vi "JSON Reponse.vi"() -> ()   [LabVIEW 2020, in "obs-scratch.lvlib"]
uses:
  obs-scratch.lvlib
  obs-websocket/GetSceneItemTransform/GetSceneItemTransform.lvclass
  C:/dev/lv20CE/relink/lv-obs-websocket/obs-websocket/Client Message/Client Message.lvclass
  obs-websocket/OBS/OBS.lvclass
  <vilib>/JDP Science/JSONtext/JSONtext.lvlib
  C:/dev/lv20CE/relink/lv-obs-websocket/obs-websocket/Request/Request.lvclass
  C:/dev/lv20CE/relink/lv-obs-websocket/obs-websocket/Message/Message.lvclass
  C:/dev/lv20CE/relink/lv-obs-websocket/obs-websocket/GetSceneItemTransform/GetSceneItemTransform.lvclass
panel:
  in  "Scale":dbl(slide) scale=0.1..5.0
  in  "Rotation":dbl min=-180.0 max=180.0 format="%0.2f"
  in  "stop":bool
  out "JSON Response":string
  out "error out":errorcluster
  in  "Password":string="44S4aN6PpCHpVM4Y"
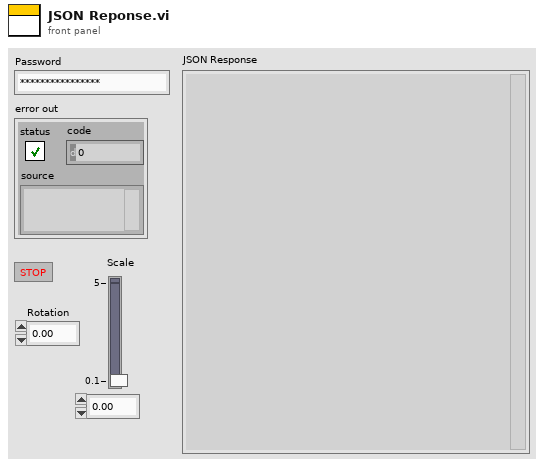
[diagram p1: front panel]
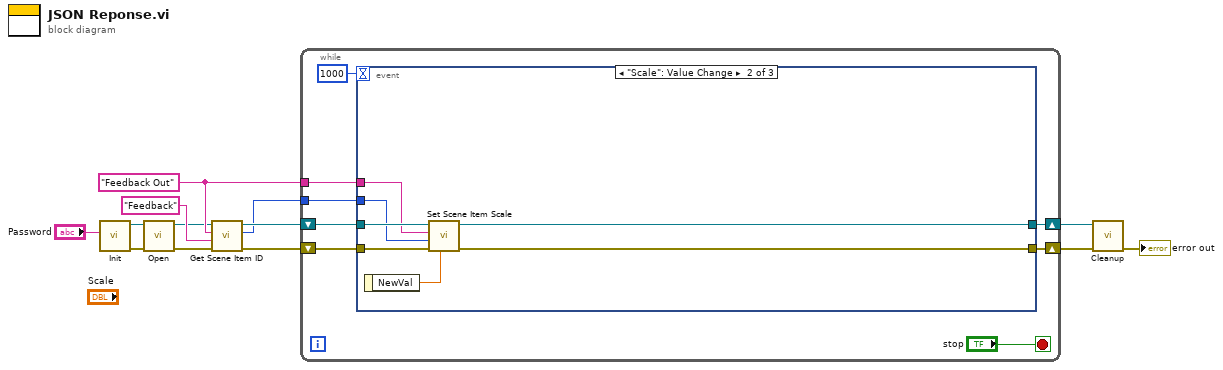
[diagram p0: block diagram]
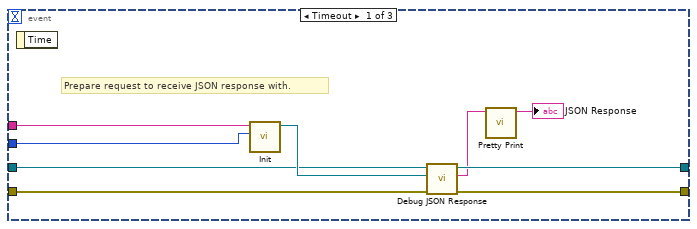
[diagram p2: hidden frame]
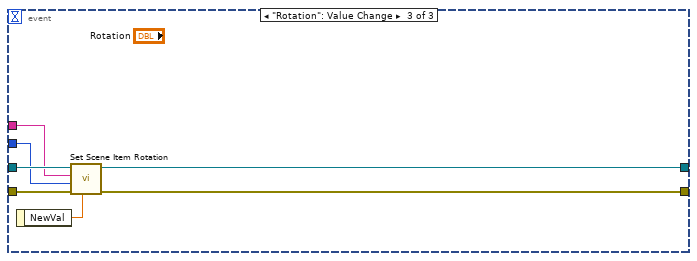
[diagram p3: hidden frame]
diagram:
  w6 = "Feedback Out" ("Scene Name")
  n1 = call "Init.vi"("Password (None)"="Password") -> ("error out"=w12:errorcluster, "OBS out"=w13:refnum<class "OBS.lvclass">)  [unwired: 9 in]
  n2 = call "Open.vi"("error in (no error)"=w12, "OBS in"=w13) -> ("error out"=w4:errorcluster, "OBS out"=w5:refnum<class "OBS.lvclass">)  [unwired: 8 in]
  n3 = call "Get Scene Item ID.vi"("error in (no error)"=w4, "Source Name"="Feedback" ("Scene Name"), "Scene Name"=w6, "OBS in"=w5) -> ("error out"=w3:errorcluster, "Scene Item ID"=w1:i32, "OBS out"=w2:refnum<class "OBS.lvclass">)  [unwired: 5 in]
  n4 = while {
    shift-right: [w18] -> w9
    shift-left: w2 -> [w21]
    shift-right: [w19] -> w10
    shift-left: w3 -> [w20]
    tunnel: w6 -> [w15]
    tunnel: w1 -> [w14]
    stop <- "stop" stop-if-true
    n5 = event shown="[1] \"Scale\": Value Change" {
      selector: _ -> [_ _ _]
      dyn-events: _ -> [_ _ _]
      timeout: 1000 -> [_ _ _]
      tunnel: w21 -> [w23 w37 w44]
      tunnel: w20 -> [w22 w36 w43]
      tunnel: [w29 w31 w38] -> w19
      tunnel: [w28 w32 w39] -> w18
      tunnel: w15 -> [w25 w33 w41]
      tunnel: w14 -> [w24 w34 w40]
      event Timeout {
        # "Prepare request to receive JSON response with."
        n6 = event-data() -> ()  [unwired: 1 in, 1 out]
        n7 = call "Init.vi"("Scene Item ID"=w24, "Scene Name"=w25) -> ("GetSceneItemTransform out"=w30:refnum<class "GetSceneItemTransform.lvclass">)  [unwired: 8 in, 1 out]
        n8 = call "Debug JSON Response.vi"("error in (no error)"=w22, "Client Message"=w30, "OBS in"=w23) -> ("error out"=w29:errorcluster, "JSON Response"=w27:string, "OBS out"=w28:refnum<class "OBS.lvclass">)  [unwired: 5 in, 1 out]
        n9 = call <vilib>:"Pretty Print.vi"("JSON"=w27) -> ("<JSON>"=→"JSON Response":string)  [unwired: 8 in, 2 out]
      }
      event "Scale": Value Change {
        n10 = event-data() -> ("NewVal"=w35:dbl)  [unwired: 1 in]
        n11 = call "Set Scene Item Scale.vi"("Scale"=w35, "error in (no error)"=w36, "Scene Item ID"=w34, "Scene Name"=w33, "OBS in"=w37) -> ("error out"=w31:errorcluster, "OBS out"=w32:refnum<class "OBS.lvclass">)  [unwired: 5 in]
      }
      event "Rotation": Value Change {
        n12 = event-data() -> ("NewVal"=w42:dbl)  [unwired: 1 in]
        n13 = call "Set Scene Item Rotation.vi"("Rotation Deg"=w42, "error in (no error)"=w43, "Scene Item ID"=w40, "Scene Name"=w41, "OBS in"=w44) -> ("error out"=w38:errorcluster, "OBS out"=w39:refnum<class "OBS.lvclass">)  [unwired: 5 in]
      }
    }
  }
  n14 = call "Cleanup.vi"("error in (no error)"=w10, "OBS in"=w9) -> ("error out"=→"error out":errorcluster)  [unwired: 9 in]
